vi "Model - Init.vi"(8 "error in (no error)":errorcluster) -> (0 "error out":errorcluster, 3 "View Model":T1)   [LabVIEW 2017]
doc: "Initialize all components of View Model"
uses:
  Controls/View Model.ctl
  Controls/Shared Model.ctl
  Error Handler/Controls/Error Model.ctl
  Error Handler/Controls/Error Event.ctl
  Error Handler/Controls/Error Type.ctl
  Controller/Controls/Controller Model.ctl
  Controller/Controls/Controller Event.ctl
  Controller/Controls/Controller Command.ctl
  Controller/Controls/Controller Overhead.ctl
  Controller/Controls/Controller Update Data.ctl
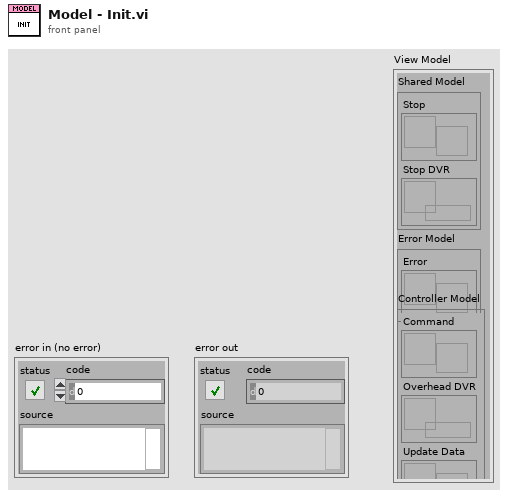
[diagram p1: front panel]
types:
  T1 = typedef "View Model.ctl" = cluster{"Shared Model":T2, "Error Model":T3, "Controller Model":T4}
  T2 = typedef "Shared Model.ctl" = cluster{"Stop":refnum<user-event>, "Stop DVR":refnum<data-value>}
  T3 = typedef "Error Model.ctl" = cluster{"Error":refnum<user-event>}
  T4 = typedef "Controller Model.ctl" = cluster{"Command":refnum<user-event>, "Overhead DVR":refnum<data-value>, "Update Data":refnum<user-event>}
  T5 = typedef "Controller Update Data.ctl" = cluster{"Blink CNTRLR2":bool, "Numeric":dbl}
  T6 = typedef "Controller Overhead.ctl" = cluster{"Start":bool, "Numeric":dbl, "Blink CNTRLR1":bool, "Blink CNTRLR2":bool}
  T7 = typedef "Controller Event.ctl" = cluster{"CMD":T8, "Data":variant}
  T8 = typedef "Controller Command.ctl" = enum16{"Idle", "Init", "Stop"}
  T9 = typedef "Error Event.ctl" = cluster{"ErrorType":T10, "error in":errorcluster}
  T10 = typedef "Error Type.ctl" = enum16{"Minor", "Critical"}
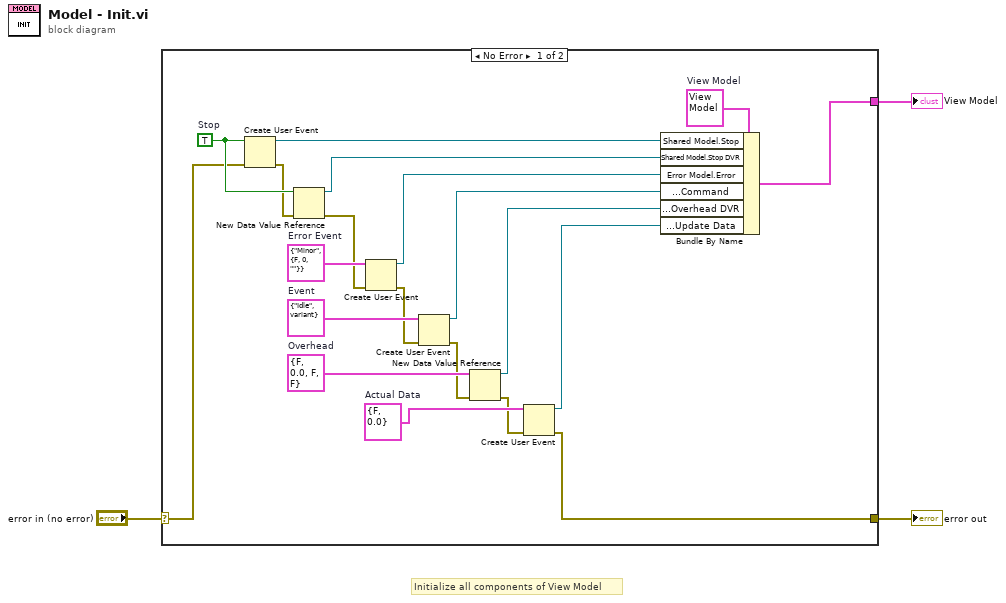
[diagram p0: block diagram]
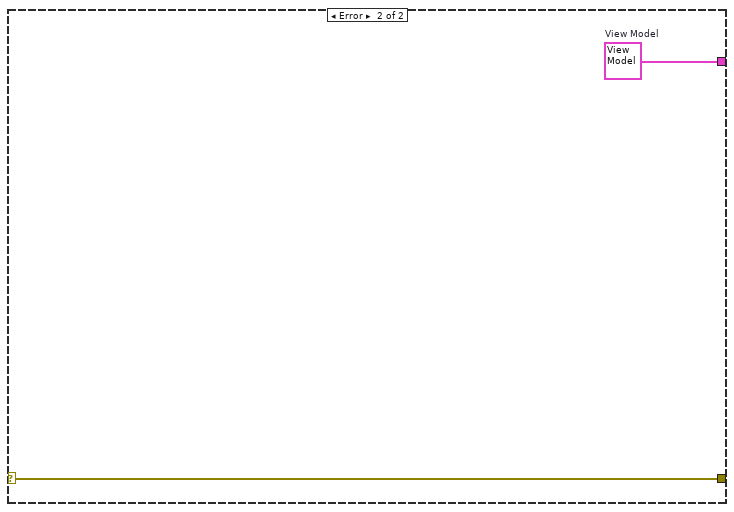
[diagram p2: hidden frame]
diagram:
  # "Initialize all components of View Model"
  n1 = case shown="No Error" "error in (no error)" {
    selector: "error in (no error)" -> [w20 w25]
    tunnel: [w4 w25] -> w2
    tunnel: [w22 w24] -> w1
    frame No Error {
      w7 = T5 {"Blink CNTRLR2"=FALSE, "Numeric"=0.0}  # Actual Data
      w14 = T6 {"Start"=FALSE, "Numeric"=0.0, "Blink CNTRLR1"=FALSE, "Blink CNTRLR2"=FALSE}  # Overhead
      w16 = T7 {"CMD"=enum."Idle", "Data"=variant}  # Event
      w18 = T9 {"ErrorType"=enum."Minor", "error in"={"status"=FALSE, "code"=0, "source"=""}}  # Error Event
      w21 = TRUE  # Stop
      w23 = T1 {"Shared Model"={"Stop"=refnum, "Stop DVR"=refnum}, "Error Model"={"Error"=refnum}, "Controller Model"={"Command"=refnum, "Overhead DVR"=refnum, "Update Data"=refnum}}  # View Model
      n2 = Create User Event(user event datatype=w21, error in=w20) -> (user event=w12:refnum<user-event>, error out=w19:errorcluster)
      n3 = New Data Value Reference(data value=w21, error in=w19) -> (data value reference=w11:refnum<data-value>, error out=w17:errorcluster)
      n4 = Create User Event(user event datatype=w18, error in=w17) -> (user event=w10:refnum<user-event>, error out=w15:errorcluster)
      n5 = Create User Event(user event datatype=w16, error in=w15) -> (user event=w9:refnum<user-event>, error out=w13:errorcluster)
      n6 = New Data Value Reference(data value=w14, error in=w13) -> (data value reference=w8:refnum<data-value>, error out=w6:errorcluster)
      n7 = Create User Event(user event datatype=w7, error in=w6) -> (user event=w5:refnum<user-event>, error out=w4:errorcluster)
      n8 = Bundle By Name(cluster=w23, "Shared Model.Stop"=w12, "Shared Model.Stop DVR"=w11, "Error Model.Error"=w10, "Controller Model.Command"=w9, "Controller Model.Overhead DVR"=w8, "Controller Model.Update Data"=w5) -> (w22:T1)
    }
    frame Error {
      w24 = T1 {"Shared Model"={"Stop"=refnum, "Stop DVR"=refnum}, "Error Model"={"Error"=refnum}, "Controller Model"={"Command"=refnum, "Overhead DVR"=refnum, "Update Data"=refnum}}  # View Model
    }
  }
  "View Model" <- w1
  "error out" <- w2
